vi "ConvertMATLABArray.vi"(1 "Array In":dbl[][](array[numeric])) -> (0 "Array Out":u8[][](array[numeric]))   [LabVIEW 2013]
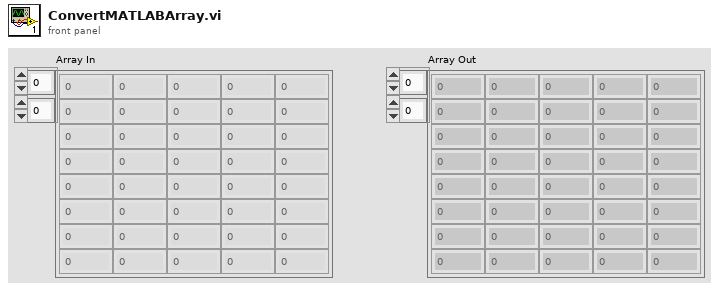
[diagram p1: front panel]
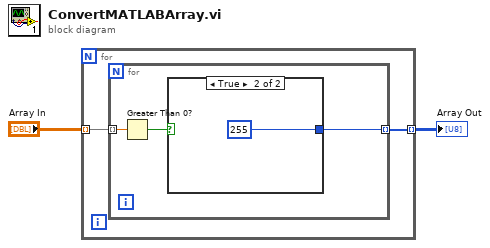
[diagram p0: block diagram]
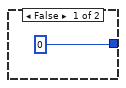
[diagram p2: hidden frame]
diagram:
  n1 = for {
    tunnel: "Array In" -> [w4] mode=indexing
    tunnel: [w3] -> w1 mode=indexing
    n2 = for {
      tunnel: w4 -> [w7] mode=indexing
      tunnel: [w5] -> w3 mode=indexing
      n3 = Greater Than 0?(x=w7) -> (x > 0?=w6:bool)
      n4 = case shown="True" w6 {
        tunnel: [u8 0 u8 255] -> w5
        frame False {
        }
        frame True {
        }
      }
    }
  }
  "Array Out" <- w1
